vi "GSP_Manager_F2_driver.vi"(4 "error in (no error)":errorcluster, 6 "Action":T1, 7 "Filter# (Move Only)":i32) -> (0 "error out":errorcluster, 3 "reference out (launch only)":refnum<vi>)   [LabVIEW 2015]
doc: "Provides an interface to the Secondary Filter Manager. See the actions below.\n\nLaunch - launch the manager thread supplying references to the controls that the thread will update.\n\nHome - Home the secondary filter\n\nMove - Move the secondary filter to the position supplied by Filter#\n\nShutdown - Shutdown the secondary filter manager"
uses:
  f2driveractions.ctl
  SystemUtil/Command.ctl
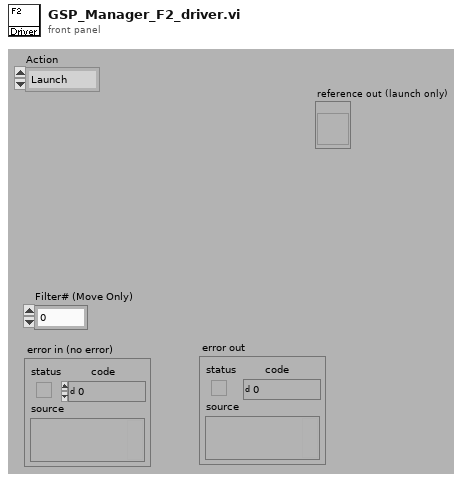
[diagram p1: front panel]
types:
  T1 = typedef "f2driveractions.ctl" = enum16{"Launch", "INIT_CTL", "Home", "Move", "Shutdown"}
  T2 = typedef "Command.ctl" = cluster{"Command":string, "Parameter":string}
  T3 = cluster{string, "type string":i16[], "data string":string}
  T4 = cluster{string, "type string":i16[], "data string":string}[]
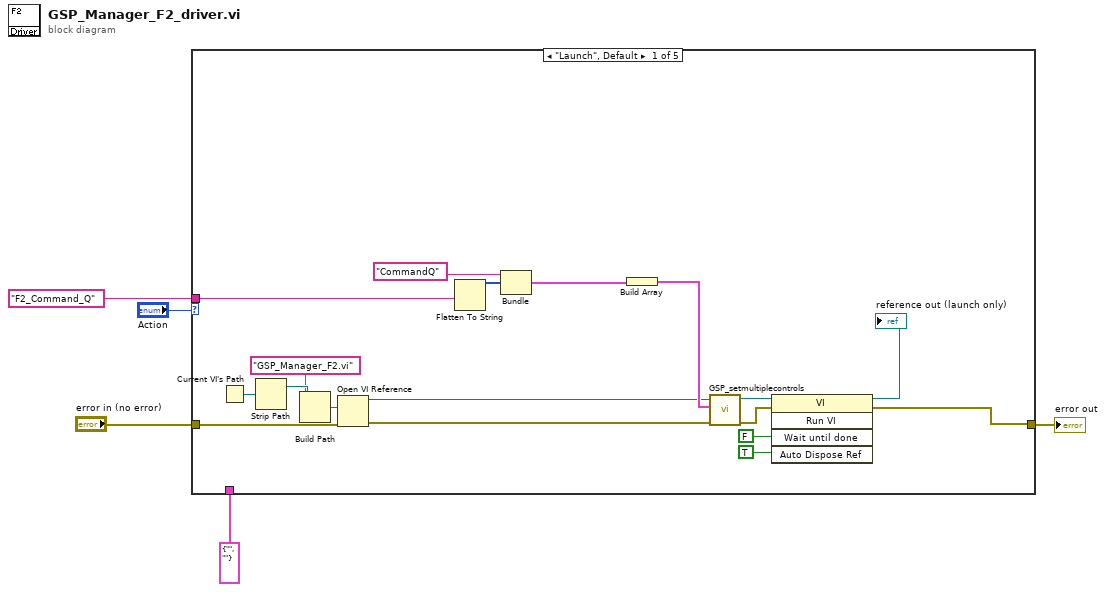
[diagram p0: block diagram]
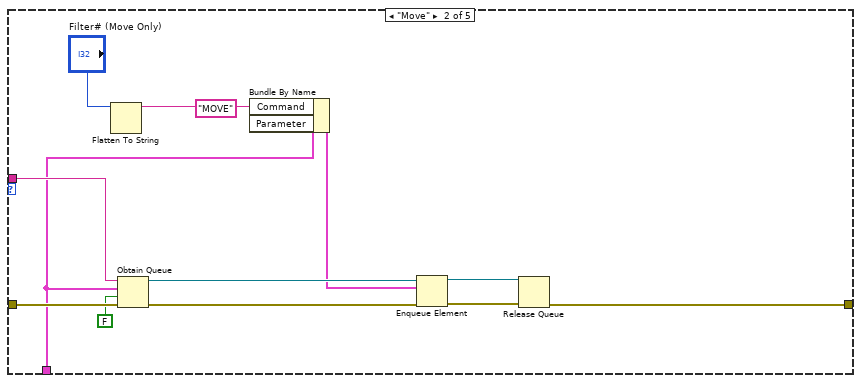
[diagram p2: hidden frame]
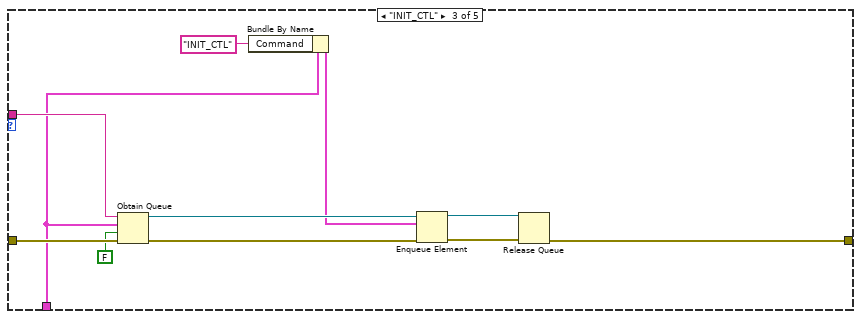
[diagram p3: hidden frame]
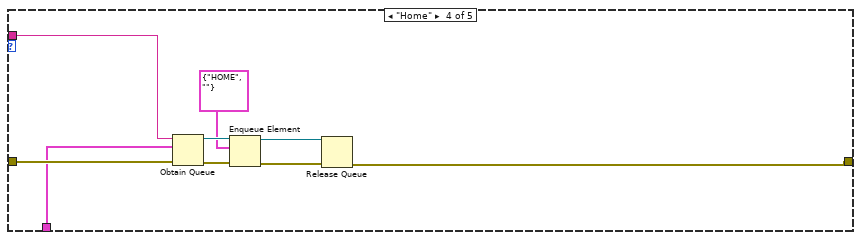
[diagram p4: hidden frame]
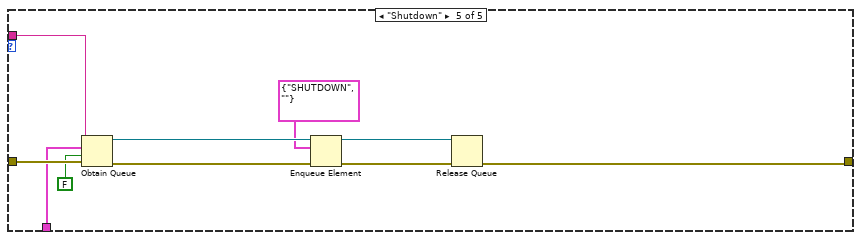
[diagram p5: hidden frame]
diagram:
  n1 = case shown="\"Launch\", Default" "Action" {
    tunnel: "error in (no error)" -> [w19 w37 w48 w55 w67]
    tunnel: [w7 w25 w38 w49 w58] -> w3
    tunnel: "F2_Command_Q" -> [w8 w36 w47 w54 w65]
    tunnel: T2 {"Command"="", "Parameter"=""} ("Command") -> [_ w32 w43 w53 w62]
    frame "Launch", Default {
      n2 = Current VI's Path() -> (path=w12:path)
      n3 = Strip Path(path=w12) -> (stripped path=w10:path)  [unwired: 1 out]
      n4 = Build Path(base path=w10, name or relative path="GSP_Manager_F2.vi" ("vi path")) -> (appended path=w11:path)
      n5 = Open VI Reference(vi path=w11, error in (no error)=w19) -> (vi reference=w17:refnum<vi>, error out=w18:errorcluster)  [unwired: 4 in]
      n6 = Flatten To String(anything=w8) -> (data string=w22:string, type string=w23:i16[])  [unwired: 3 in, 1 out]
      n7 = Bundle("CommandQ", "type string"=w23, "data string"=w22) -> (w21:T3)  [unwired: 1 in]
      n8 = Build Array(w21) -> (w20:T4)
      n9 = call "GSP_setmultiplecontrols.vi"("error in (no error)"=w18, "Control Infos"=w20, "reference"=w17) -> ("error out"=w15:errorcluster, "reference out"=w16:refnum<vi>)  [unwired: 3 in]
      n10 = invoke class="VI" method="Run VI"(reference=w16, error in=w15, "Wait until done"=FALSE, "Auto Dispose Ref"=TRUE) -> (reference out=→"reference out (launch only)":refnum<vi>, error out=w7:errorcluster)  [unwired: 1 in, 3 out]
    }
    frame "Move" {
      n11 = Flatten To String(anything="Filter# (Move Only)") -> (data string=w28:string)  [unwired: 3 in, 2 out]
      n12 = Obtain Queue(name (unnamed)=w36, element data type=w32, create if not found? (T)=FALSE, error in (no error)=w37) -> (queue out=w35:refnum<queue>, error out=w34:errorcluster)  [unwired: 1 in, 1 out]
      n13 = Bundle By Name(cluster=w32, "Command"="MOVE" ("element"), "Parameter"=w28) -> (w30:T2)
      n14 = Enqueue Element(queue=w35, element=w30, error in (no error)=w34) -> (queue out=w27:refnum<queue>, error out=w26:errorcluster)  [unwired: 1 in, 1 out]
      n15 = Release Queue(queue=w27, error in (no error)=w26) -> (error out=w25:errorcluster)  [unwired: 1 in, 2 out]
    }
    frame "INIT_CTL" {
      n16 = Obtain Queue(name (unnamed)=w47, element data type=w43, create if not found? (T)=FALSE, error in (no error)=w48) -> (queue out=w46:refnum<queue>, error out=w45:errorcluster)  [unwired: 1 in, 1 out]
      n17 = Bundle By Name(cluster=w43, "Command"="INIT_CTL" ("element")) -> (w41:T2)
      n18 = Enqueue Element(queue=w46, element=w41, error in (no error)=w45) -> (queue out=w40:refnum<queue>, error out=w39:errorcluster)  [unwired: 1 in, 1 out]
      n19 = Release Queue(queue=w40, error in (no error)=w39) -> (error out=w38:errorcluster)  [unwired: 1 in, 2 out]
    }
    frame "Home" {
      n20 = Obtain Queue(name (unnamed)=w54, element data type=w53, error in (no error)=w55) -> (queue out=w57:refnum<queue>, error out=w56:errorcluster)  [unwired: 2 in, 1 out]
      n21 = Enqueue Element(queue=w57, element=T2 {"Command"="HOME", "Parameter"=""}, error in (no error)=w56) -> (queue out=w51:refnum<queue>, error out=w50:errorcluster)  [unwired: 1 in, 1 out]
      n22 = Release Queue(queue=w51, error in (no error)=w50) -> (error out=w49:errorcluster)  [unwired: 1 in, 2 out]
    }
    frame "Shutdown" {
      n23 = Obtain Queue(name (unnamed)=w65, element data type=w62, create if not found? (T)=FALSE, error in (no error)=w67) -> (queue out=w64:refnum<queue>, error out=w66:errorcluster)  [unwired: 1 in, 1 out]
      n24 = Enqueue Element(queue=w64, element=T2 {"Command"="SHUTDOWN", "Parameter"=""}, error in (no error)=w66) -> (queue out=w60:refnum<queue>, error out=w59:errorcluster)  [unwired: 1 in, 1 out]
      n25 = Release Queue(queue=w60, error in (no error)=w59) -> (error out=w58:errorcluster)  [unwired: 1 in, 2 out]
    }
  }
  "error out" <- w3
